vi "Car Wash System Globals.vi"() -> ()   [LabVIEW 2017]
doc: "This global variable contains all of the strings that are displayed to the user interface or logged to disk by the BoilerMain application."
panel:
  out "Bug Remover":string="Bug Remover"
  out "Under Body Wash":string="Under Body Wash"
  out "Air Dry":string="Air Dry"
  out "Tire Shine Foam":string="Tire Shine Foam"
  out "Spot Free Rinse":string="Spot Free Rinse"
  out "Low Pressure Wax":string="Low Pressure Wax"
  out "High Pressure Wash":string="High Pressure Wash"
  out "Pre-Soak":string="Pre-Soak"
  out "Configuration Files":string="Configuration Files"
  out "Enter Filename:":string="Select a Boiler INI File:"
  out "Controller":string="Controller"
  out "Error Logged":string="A critical error occurred.  Check Error Log.txt for more information."
  out "VI Stopped":string="VI Stopped"
  out "True":string="True"
  out "Event":string="Event"
  out "Event Data":string="Event Data"
  out "Timestamp":string="Timestamp"
  out "Lockout":string="Lockout"
  # "Status Log Headers"
  # "INI File Strings"
  # "Constants"
  # "Status Strings"
  # "Error Logging"
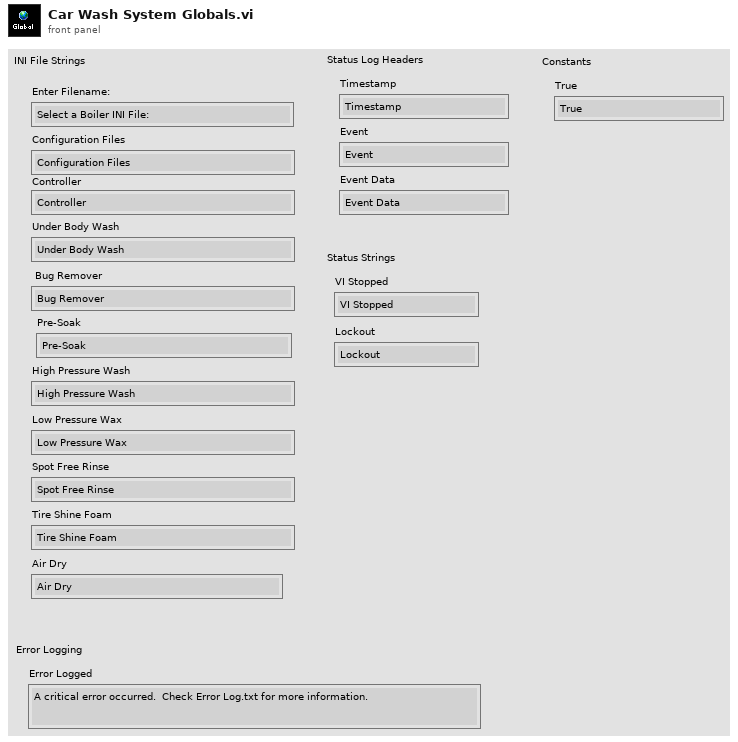
[diagram p1: front panel]
diagram:
